vi "close MB.vi"(8 "Error in":errorcluster caption="Error in (no error)") -> (0 "error out":errorcluster)   [LabVIEW 2016, in "环境动力监测库.lvlib" / "浮标电源管理.lvlib"]
uses:
  <vilib>/Plasmionique/MB Master/MB_Master/MB_Master.lvclass
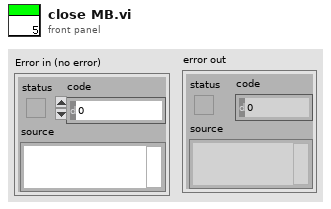
[diagram p1: front panel]
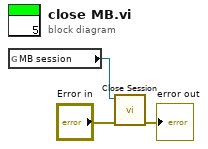
[diagram p0: block diagram]
diagram:
  n1 = global read "通讯全局变量.vi" "MB session"() -> (w2:refnum<class "MB_Master.lvclass">)
  n2 = call-dynamic "Close Session.vi"("error in (no error)"="Error in", "MB session in"=w2) -> ("error out"=→"error out":errorcluster)  [unwired: 9 in]
